vi "validate line configuration.vi"(7 "Module Config":refnum<class "Sequencer Module configuration.lvclass">, 11 "Mappings in":T1) -> (1 "valid?":bool, 2 "errors":string, 3 "Mappings out":T1)   [LabVIEW 2015, in "Sequencer Module editor node.lvclass"]
doc: "This VI validates modifications to the table of lines and returns any errors as strings."
uses:
  Sequencer Module editor node.lvclass
  Mappings.ctl
  <vilib>/NI/Tag Bus Module Framework/channel/TBM channel.lvclass
  classes/Sequence/Config/Sequence Config.lvclass
  module/configuration/Line.ctl
  Map.ctl
  module/configuration/Sequencer Module configuration.lvclass
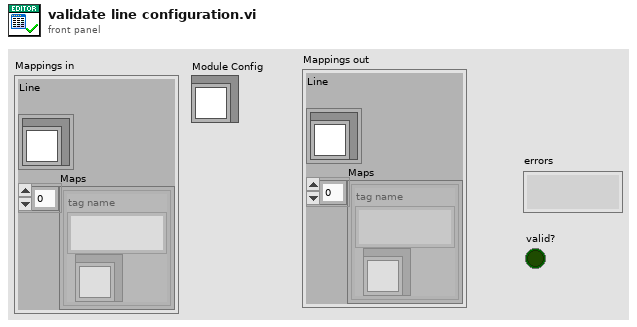
[diagram p1: front panel]
types:
  T1 = typedef "Sequencer Module editor node.lvclass/Mappings.ctl" = cluster{"Line":T2, "Maps":T3[]}
  T2 = typedef "Sequencer Module configuration.lvclass/Line.ctl" = cluster{"Sequence":refnum<class "Sequence Config.lvclass">}
  T3 = typedef "Sequencer Module editor node.lvclass/Map.ctl" = cluster{"channel":refnum<class "TBM channel.lvclass">, "tag name":string}
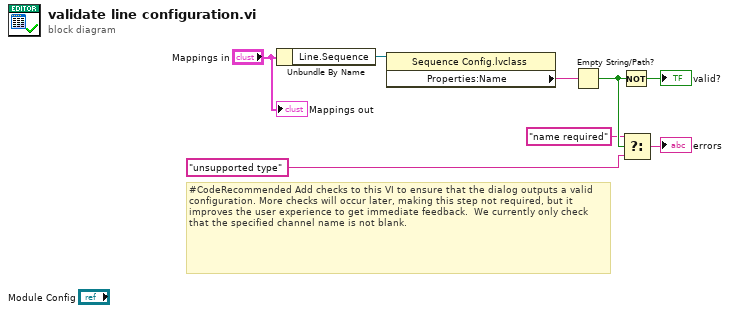
[diagram p0: block diagram]
diagram:
  # "#CodeRecommended Add checks to this VI to ensure that the dialog outputs a valid configuration. More checks will occur later, making this step not required, but it improves the user experience to get immediate feedback.  We currently only check that the specified channel name is not blank."
  n1 = Unbundle By Name("Mappings in") -> ("Line.Sequence"=w7:refnum<class "Sequence Config.lvclass">)
  n2 = property class="Sequence Config.lvclass"(reference=w7) -> ("Properties:Name"=w6:string)  [unwired: 1 in, 2 out]
  n3 = Empty String/Path?(string/path=w6) -> (empty?=w4:bool)
  n4 = Not(x=w4) -> (.not. x?=→"valid?":bool)
  n5 = Select(t="name required", s=w4, f="unsupported type") -> (s? t:f=→"errors":string)
  "Mappings out" <- "Mappings in"
